vi "140117-Interpolate_image_subregion-SubVI.vi"(4 "Image":u16[][](array[numeric]), 6 "y fit position":dbl, 7 "Mask":dbl[][](array[numeric]), 9 "x fit position":dbl, 10 "sub region width":dbl, 11 "Interp. multip.":i32) -> (1 "Sub Image":u16[][](array[numeric]), 2 "Array":dbl[][](array[numeric]), 3 "Avg. in area":dbl, 5 "Masked region":dbl[][](array[numeric]))   [LabVIEW 2012]
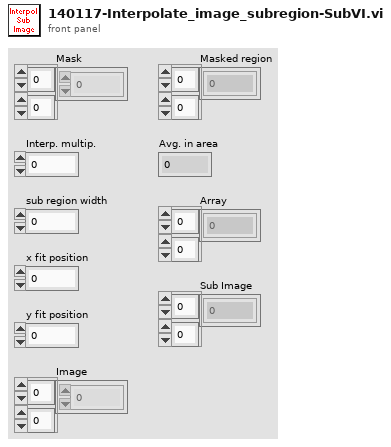
[diagram p1: front panel]
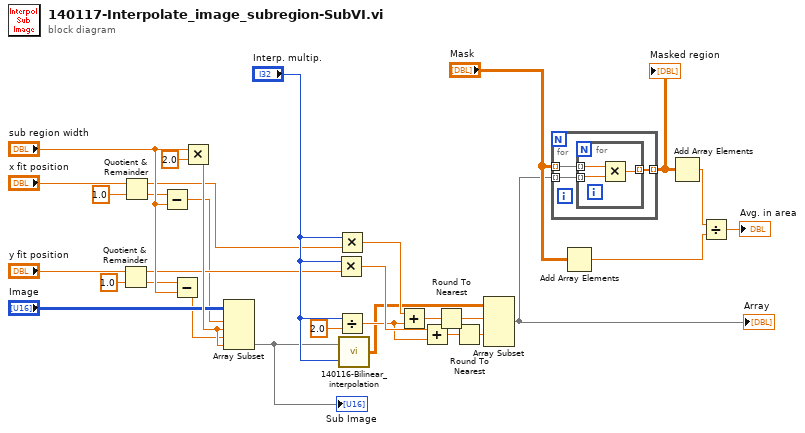
[diagram p0: block diagram]
diagram:
  n1 = Quotient & Remainder(x="y fit position", y=1.0) -> (x-y*floor(x/y)=w13:dbl, floor(x/y)=w12:dbl)
  n2 = Quotient & Remainder(x="x fit position", y=1.0) -> (x-y*floor(x/y)=w8:dbl, floor(x/y)=w10:dbl)
  n3 = Subtract(x=w10, y="sub region width") -> (x-y=w1:dbl)
  n4 = Subtract(x=w12, y="sub region width") -> (x-y=w2:dbl)
  n5 = Multiply(x="sub region width", y=2.0) -> (x*y=w16:dbl)
  n6 = Array Subset(array="Image", index (row)=w1, length (row)=w16, index (col)=w2, length (col)=w16) -> (w4:u16[][])
  "Sub Image" <- w4
  n7 = Multiply(x="Interp. multip.", y=w13) -> (x*y=w24:dbl)
  n8 = Multiply(x="Interp. multip.", y=w8) -> (x*y=w19:dbl)
  n9 = Divide(x="Interp. multip.", y=2.0) -> (x/y=w23:dbl)
  n10 = call "140116-Bilinear_interpolation.vi"("multiplier"="Interp. multip.", "Array"=w4) -> ("10x Bilinear interpolation"=w7:dbl[][])
  n11 = Add(x=w19, y=w23) -> (x+y=w20:dbl)
  n12 = Add(x=w24, y=w23) -> (x+y=w22:dbl)
  n13 = Round To Nearest(number=w20) -> (nearest integer value=w21:dbl)
  n14 = Round To Nearest(number=w22) -> (nearest integer value=w14:dbl)
  n15 = Array Subset(array=w7, index (row)=w21, index (col)=w14) -> (w27:dbl[][])  [unwired: 2 in]
  "Array" <- w27
  n16 = for {
    tunnel: "Mask" -> [w34] mode=indexing
    tunnel: w27 -> [w33] mode=indexing
    tunnel: [w32] -> w26 mode=indexing
    n17 = for {
      tunnel: w34 -> [w36] mode=indexing
      tunnel: w33 -> [w37] mode=indexing
      tunnel: [w35] -> w32 mode=indexing
      n18 = Multiply(x=w36, y=w37) -> (x*y=w35:dbl)
    }
  }
  "Masked region" <- w26
  n19 = Add Array Elements(numeric array="Mask") -> (sum=w28:dbl)
  n20 = Add Array Elements(numeric array=w26) -> (sum=w29:dbl)
  n21 = Divide(x=w29, y=w28) -> (x/y=→"Avg. in area":dbl)
